vi "Robot Global Data.vi"() -> ()   [LabVIEW 2017]
doc: "This global VI can contain as many global variables as you need. Place a control on the panel, give it a good name. To read or write to it from a VI, drag the icon to the diagram of that VI. You can also drag from the project. Click on the node to change which global you access. You shouldn't have multiple locations writing to a global or it will cause a race-condition."
uses:
  <vilib>/Rock Robotics/WPI/Camera/WPI_CameraImageSize.ctl
  <vilib>/Rock Robotics/WPI/DriverStation/WPI_DriverStationRobotMode2.ctl
panel:
  in  "Stop Command?":bool
  in  "Reset Gyro?":bool
  in  "Jog Mode":T1
  in  "Invert Drive?":bool
  in  "Shooter RPM":dbl
  in  "Ultrasonic Distance":dbl
  in  "YRPHfH":T2
  in  "Robot Mode":T3
  in  "image size":T4=enum."320x240"
  in  "Enable Vision":bool
  # "FRC Team 34 Global Data"
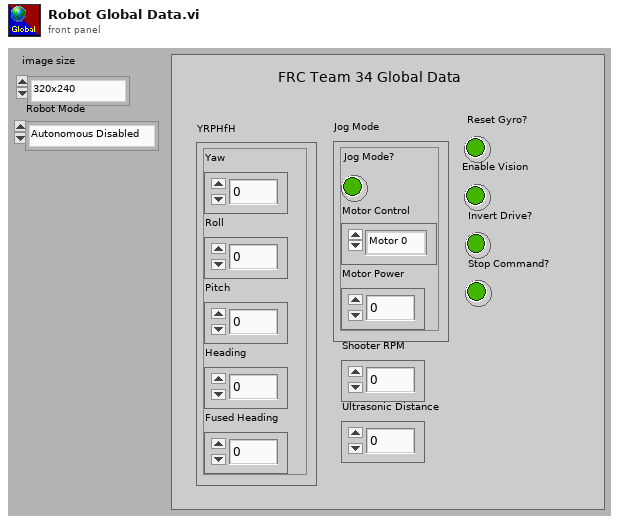
[diagram p1: front panel]
types:
  T1 = cluster{"Jog Mode?":bool, "Motor Control":enum16{"Motor 0", "Motor 1", "Motor 2", "Motor 3", "Motor 4", "Motor 5", "Motor 6", "Motor 7"}, "Motor Power":dbl}
  T2 = cluster{"Yaw":dbl, "Roll":dbl, "Pitch":dbl, "Heading":dbl, "Fused Heading":dbl}
  T3 = typedef "WPI_DriverStationRobotMode2.ctl" = enum16{"Autonomous Disabled", "Autonomous Enabled", "Teleop Disabled", "Teleop Enabled", "Disconnected", "Finish", "Test Disabled", "Test Enabled", "Emergency Stopped"}
  T4 = typedef "WPI_CameraImageSize.ctl" = enum16{"640x480", "320x240", "160x120", "Custom"}
diagram:
